vi "MultiScanXPS.vi"() -> ()   [LabVIEW 2016]
panel:
  in  "V Range 2":dbl
  in  "Initial V 2":dbl
  out "I/V Curve 2":cluster{"X":dbl[], "Y":dbl[]}[](graph) caption="XY Graph"
  out "Current 2":dbl format="%0.2f"
  out "Voltage 2":dbl format="%0.2f"
  in  "Range/N = dV":i32
  in  "Repeats":i32=10
  in  "Filename":path=path "C:/Users/tysoe-lab/Desktop/1.lvm"
  in  "Comment":string
  in  "V Range":dbl
  in  "Initial V":dbl
  in  "Number of samples":i32=10
  out "I/V Curve":cluster{"X":dbl[], "Y":dbl[]}[](graph) caption="XY Graph"
  out "Current":dbl format="%0.2f"
  out "Voltage":dbl format="%0.2f"
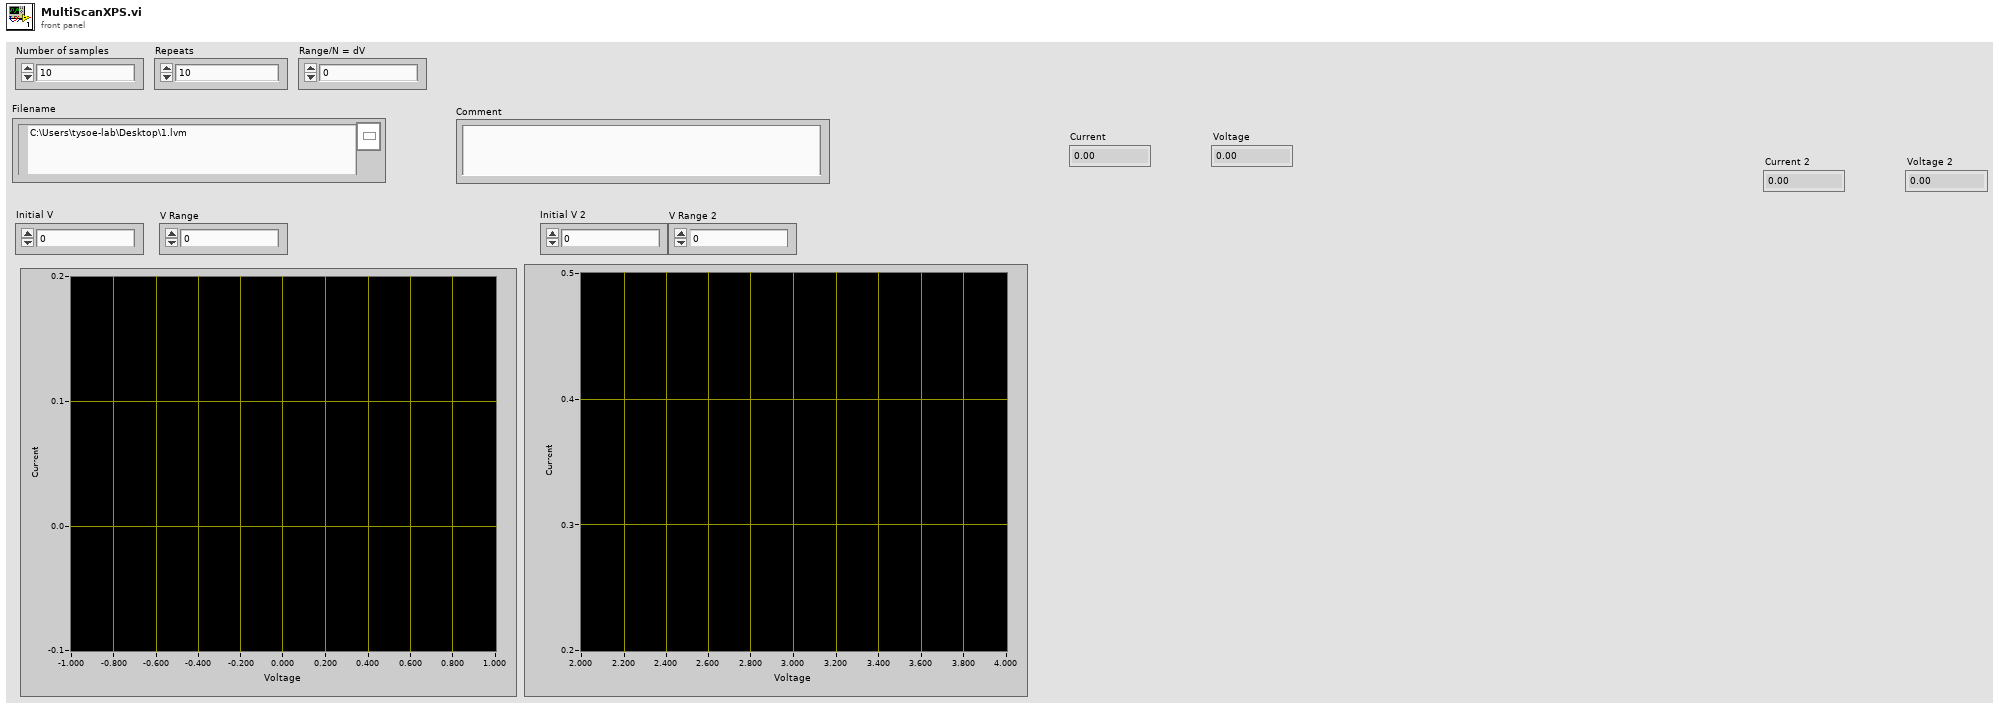
[diagram p1: front panel]
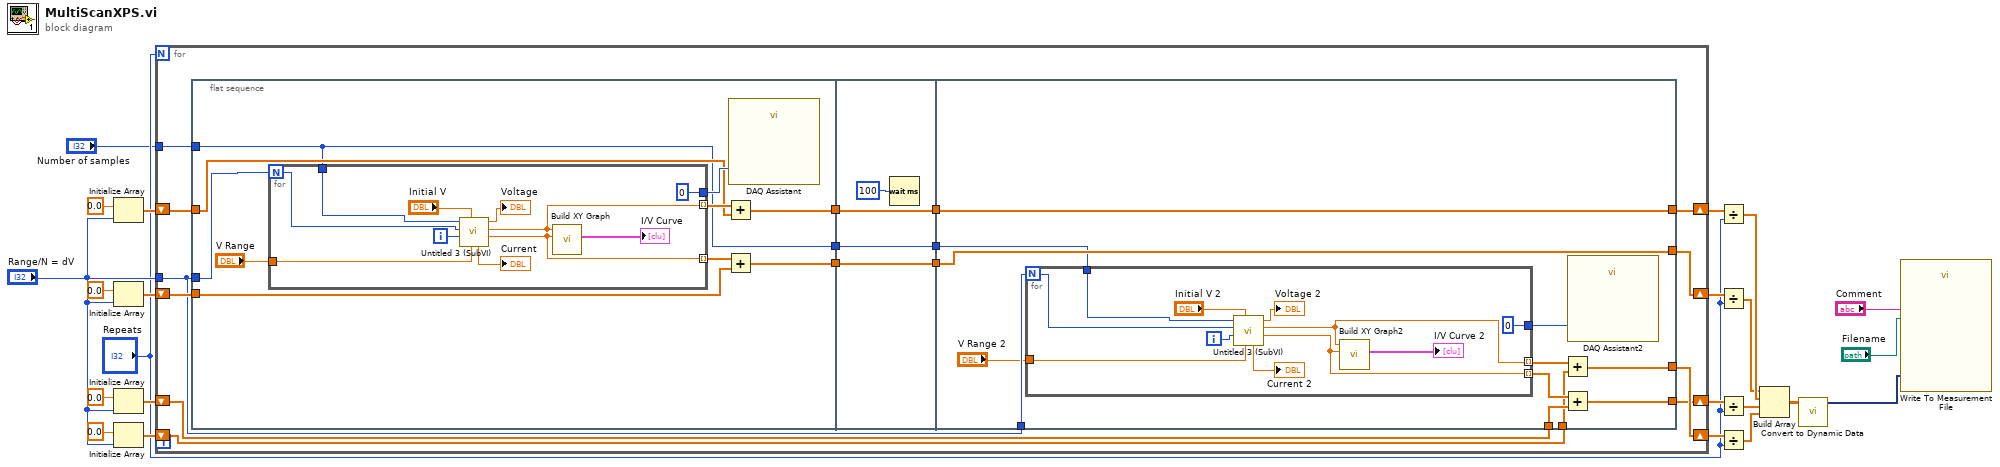
[diagram p0: block diagram]
diagram:
  n1 = Initialize Array(0.0 ("element"), "Range/N = dV") -> (w15:dbl[])
  n2 = Initialize Array(0.0 ("element"), "Range/N = dV") -> (w23:dbl[])
  n3 = Initialize Array(0.0 ("element"), "Range/N = dV") -> (w10:dbl[])
  n4 = Initialize Array(0.0 ("element"), "Range/N = dV") -> (w9:dbl[])
  n5 = for {
    N: "Repeats" -> [_]
    shift-right: [w38] -> w18
    shift-left: w23 -> [w39]
    shift-right: [w36] -> w14
    shift-left: w15 -> [w37]
    tunnel: "Range/N = dV" -> [w31]
    shift-right: [w27] -> w7
    shift-left: w10 -> [w30]
    shift-right: [w28] -> w8
    shift-left: w9 -> [w29]
    tunnel: "Number of samples" -> [w26]
    n6 = flat-sequence {
      tunnel: w39 -> [w47]
      tunnel: w37 -> [w43]
      tunnel: w31 -> [w41]
      tunnel: [w45] -> w35
      tunnel: [w42] -> w34
      tunnel: w26 -> [w40]
      tunnel: [w40] -> w24
      tunnel: w35 -> [w64]
      tunnel: w34 -> [w63]
      tunnel: [w64] -> w33
      tunnel: [w63] -> w32
      tunnel: [w61] -> w25
      tunnel: w24 -> [w61]
      tunnel: [w75] -> w36
      tunnel: [w76] -> w38
      tunnel: w33 -> [w76]
      tunnel: w32 -> [w75]
      tunnel: w31 -> [w71]
      tunnel: w30 -> [w70]
      tunnel: w29 -> [w69]
      tunnel: [w68] -> w28
      tunnel: [w67] -> w27
      tunnel: w25 -> [w65]
      frame #0 {
        n7 = for {
          N: w41 -> [w57]
          tunnel: "V Range" -> [w59]
          tunnel: [w55] -> w46 mode=indexing
          tunnel: [w53] -> w44 mode=indexing
          tunnel: [0] -> w48
          tunnel: w40 -> [w50]
          i -> [w58]
          n8 = call "Untitled 3 (SubVI).vi"("V Range"=w59, "Initial V"="Initial V", "Numeric 3"=w58, "Numeric in"=w57, "Number of samples"=w50) -> ("mean"=w55:dbl, "Numeric out"=w53:dbl, "Voltage"=→"Voltage":dbl, "Current"=→"Current":dbl)  [unwired: 3 in]
          n9 = call "Build XY Graph"("Y Input"=w55, "X Input"=w53) -> ("XY Graph"=→"I/V Curve":cluster{"X":dbl[], "Y":dbl[]}[])  [unwired: 8 in, 1 out]
        }
        n10 = Add(x=w44, y=w43) -> (x+y=w42:dbl[])
        n11 = Add(x=w46, y=w47) -> (x+y=w45:dbl[])
        n12 = call "DAQ Assistant"("data"=w48) -> ()  [unwired: 17 in, 2 out]
      }
      frame #1 {
        n13 = Wait (ms)(milliseconds to wait=u32 100) -> ()  [unwired: 1 out]
      }
      frame #2 {
        n14 = for {
          N: w71 -> [w84]
          tunnel: "V Range 2" -> [w86]
          tunnel: [w82] -> w73 mode=indexing
          tunnel: [w80] -> w72 mode=indexing
          tunnel: [0] -> w74
          tunnel: w65 -> [w77]
          i -> [w85]
          n15 = call "Untitled 3 (SubVI).vi"("V Range"=w86, "Initial V"="Initial V 2", "Numeric 3"=w85, "Numeric in"=w84, "Number of samples"=w77) -> ("mean"=w82:dbl, "Numeric out"=w80:dbl, "Voltage"=→"Voltage 2":dbl, "Current"=→"Current 2":dbl)  [unwired: 3 in]
          n16 = call "Build XY Graph2"("Y Input"=w82, "X Input"=w80) -> ("XY Graph"=→"I/V Curve 2":cluster{"X":dbl[], "Y":dbl[]}[])  [unwired: 8 in, 1 out]
        }
        n17 = Add(x=w72, y=w69) -> (x+y=w68:dbl[])
        n18 = Add(x=w73, y=w70) -> (x+y=w67:dbl[])
        n19 = call "DAQ Assistant2"("data"=w74) -> ()  [unwired: 17 in, 2 out]
      }
    }
  }
  n20 = Divide(x=w14, y="Repeats") -> (x/y=w2:dbl[])
  n21 = Divide(x=w18, y="Repeats") -> (x/y=w1:dbl[])
  n22 = Divide(x=w7, y="Repeats") -> (x/y=w6:dbl[])
  n23 = Divide(x=w8, y="Repeats") -> (x/y=w5:dbl[])
  n24 = Build Array(w1, w2, w6, w5) -> (w19:dbl[][])
  n25 = call "Convert to Dynamic Data"("2D Array"=w19) -> ("Dynamic Data Type"=w22:dynamicdata)  [unwired: 3 in]
  n26 = call "Write To Measurement File"("Signals"=w22, "Filename"="Filename", "Comment"="Comment") -> ()  [unwired: 14 in, 3 out]
